vi "test_easy_spline_fft.vi"() -> ()   [LabVIEW 2009]
doc: "Copyright (c) 2010 Stepan A. Baranov (stepan@baranov.su)\nAll rights reserved.\nweb-site: www.OCTLab.org"
uses:
  <vilib>/Analysis/4window.llb/Hanning Window (DBL).vi
  <vilib>/Analysis/NI_AALPro.lvlib
  OCTLib_64.dll
panel:
  out "error out":errorcluster
  out "Im part":dbl[](array[numeric])
  out "Re part":dbl[](array[numeric])
  out "Phase A-scan":dbl[](array[numeric])
  out "Intensity A-scan":dbl[](array[numeric])
  out "Im":dbl[](array[numeric])
  out "Re":dbl[](array[numeric])
  out "phase":dbl[](array[numeric])
  out "intensity":dbl[](array[numeric])
  out "time for FFT":u32
  in  "RSM_STAT?":bool=TRUE
  in  "stop":bool
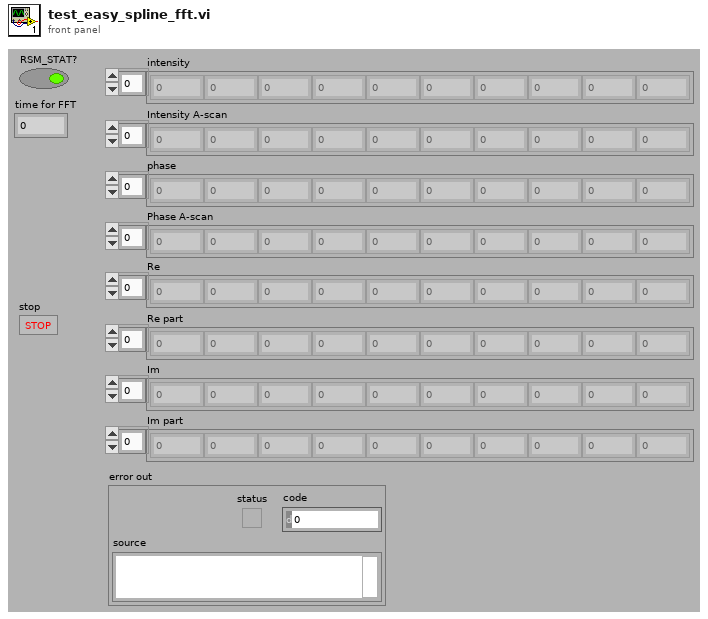
[diagram p1: front panel]
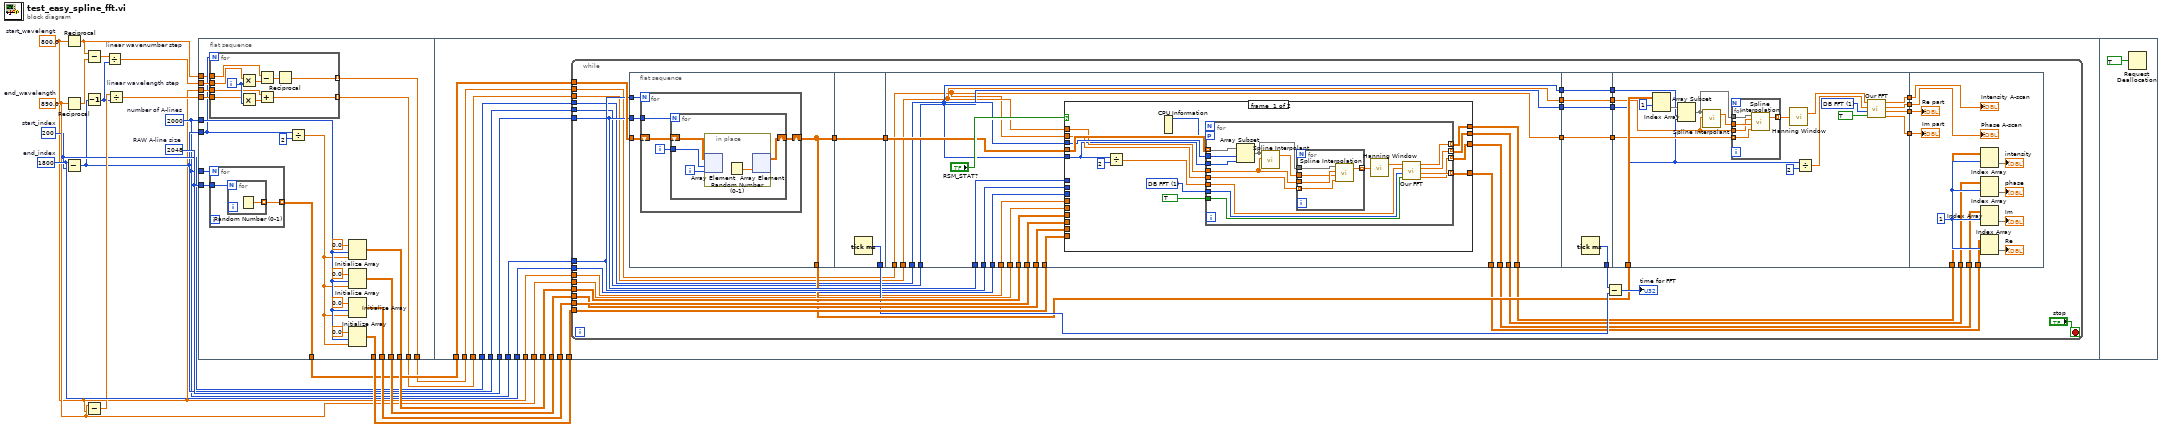
[diagram p0: block diagram]
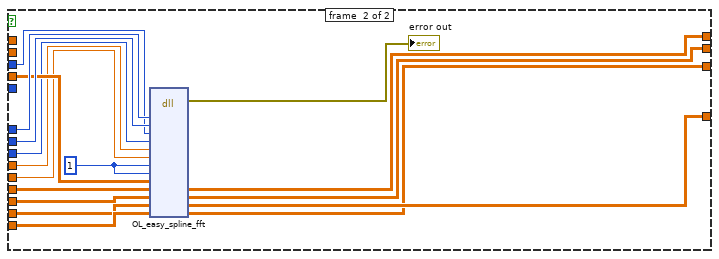
[diagram p2: hidden frame]
diagram:
  w1 = 800.0  # start_wavelengt
  w9 = 890.0  # end_wavelength
  w15 = 1800  # end_index
  w8 = 200  # start_index
  w4 = 2000  # number of A-lines
  w16 = 2048  # RAW A-line size
  n1 = Reciprocal(x=w1) -> (1/x=w2:dbl)
  n2 = Reciprocal(x=w9) -> (1/x=w3:dbl)
  n3 = Subtract(x=w15, y=w8) -> (x-y=w7:i32)
  n4 = Subtract(x=w2, y=w3) -> (x-y=w13:dbl)
  n5 = Decrement(x=w7) -> (x-1=w12:i32)
  n6 = Subtract(x=w9, y=w1) -> (x-y=w14:dbl)
  n7 = Divide "linear wavenumber step"(x=w13, y=w12) -> (x/y=w11:dbl)
  n8 = Divide "linear wavelength step"(x=w14, y=w12) -> (x/y=w10:dbl)
  n9 = flat-sequence {
    tunnel: w16 -> [w42]
    tunnel: w4 -> [w41]
    tunnel: w4 -> [w36]
    tunnel: [w35] -> w21
    tunnel: [w34] -> w20
    tunnel: [w33] -> w19
    tunnel: [w32] -> w18
    tunnel: [w31] -> w17
    tunnel: w7 -> [w25]
    tunnel: w11 -> [w30]
    tunnel: w10 -> [w29]
    tunnel: w1 -> [w28]
    tunnel: [w27] -> w6
    tunnel: [w26] -> w5
    tunnel: w2 -> [w22]
    tunnel: w4 -> [w69]
    tunnel: w16 -> [w68]
    tunnel: w21 -> [w67]
    tunnel: w20 -> [w66]
    tunnel: w19 -> [w65]
    tunnel: w18 -> [w64]
    tunnel: w17 -> [w63]
    tunnel: w8 -> [w62]
    tunnel: w15 -> [w61]
    tunnel: w1 -> [w60]
    tunnel: w9 -> [w59]
    tunnel: w7 -> [w58]
    tunnel: w6 -> [w57]
    tunnel: w5 -> [w56]
    frame #0 {
      n10 = for {
        N: w25 -> [_]
        tunnel: w30 -> [w52]
        tunnel: [w44] -> w26 mode=indexing
        tunnel: w29 -> [w49]
        tunnel: w28 -> [w48]
        tunnel: [w43] -> w27 mode=indexing
        tunnel: w22 -> [w46]
        i -> [w50]
        n11 = Multiply(x=w52, y=w50) -> (x*y=w51:dbl)
        n12 = Multiply(x=w49, y=w50) -> (x*y=w47:dbl)
        n13 = Subtract(x=w46, y=w51) -> (x-y=w45:dbl)
        n14 = Add(x=w48, y=w47) -> (x+y=w43:dbl)
        n15 = Reciprocal(x=w45) -> (1/x=w44:dbl)
      }
      n16 = for {
        N: w41 -> [_]
        tunnel: [w54] -> w31 mode=indexing
        tunnel: w42 -> [w53]
        n17 = for {
          N: w53 -> [_]
          tunnel: [w55] -> w54 mode=indexing
          n18 = Random Number (0-1)() -> (number: 0 to 1=w55:dbl)
        }
      }
      n19 = Divide(x=w25, y=2) -> (x/y=w23:dbl)
      n20 = Initialize Array(0.0 ("element"), w36, w23) -> (w34:dbl[][])
      n21 = Initialize Array(0.0 ("element"), w36, w23) -> (w33:dbl[][])
      n22 = Initialize Array(0.0 ("element"), w36, w23) -> (w35:dbl[][])
      n23 = Initialize Array(0.0 ("element"), w36, w23) -> (w32:dbl[][])
    }
    frame #1 {
      n24 = while {
        tunnel: w63 -> [w105]
        tunnel: w69 -> [w97]
        tunnel: w68 -> [w96]
        tunnel: w67 -> [w104]
        tunnel: w66 -> [w103]
        tunnel: w65 -> [w102]
        tunnel: w64 -> [w101]
        tunnel: w62 -> [w84]
        tunnel: w61 -> [w83]
        tunnel: w60 -> [w82]
        tunnel: w59 -> [w81]
        tunnel: w58 -> [w80]
        tunnel: w57 -> [w79]
        tunnel: w56 -> [w78]
        stop <- "stop" stop-if-true
        n25 = flat-sequence {
          tunnel: w105 -> [w110]
          tunnel: w97 -> [w109]
          tunnel: w96 -> [w108]
          tunnel: [w107] -> w95
          tunnel: [w107] -> w85
          tunnel: [w121] -> w100
          tunnel: [w120] -> w86
          tunnel: w85 -> [w120]
          tunnel: w104 -> [w139]
          tunnel: w103 -> [w138]
          tunnel: w102 -> [w137]
          tunnel: w101 -> [w136]
          tunnel: w96 -> [w135]
          tunnel: w97 -> [w134]
          tunnel: [w133] -> w90
          tunnel: [w132] -> w89
          tunnel: [w131] -> w88
          tunnel: [w130] -> w87
          tunnel: w86 -> [w129]
          tunnel: w84 -> [w125]
          tunnel: w83 -> [w128]
          tunnel: w82 -> [w127]
          tunnel: w81 -> [w126]
          tunnel: w80 -> [w124]
          tunnel: w79 -> [w123]
          tunnel: w78 -> [w122]
          tunnel: [w125] -> w76
          tunnel: [w124] -> w74
          tunnel: [w123] -> w73
          tunnel: [w122] -> w70
          tunnel: [w197] -> w98
          tunnel: [w196] -> w77
          tunnel: w76 -> [w196]
          tunnel: [w195] -> w75
          tunnel: w74 -> [w195]
          tunnel: w73 -> [w194]
          tunnel: [w194] -> w72
          tunnel: [w193] -> w71
          tunnel: w70 -> [w193]
          tunnel: w95 -> [w216]
          tunnel: [w211] -> w94
          tunnel: [w210] -> w93
          tunnel: [w209] -> w92
          tunnel: [w208] -> w91
          tunnel: w77 -> [w205]
          tunnel: w75 -> [w200]
          tunnel: w72 -> [w203]
          tunnel: w71 -> [w202]
          tunnel: w94 -> [w234]
          tunnel: w93 -> [w233]
          tunnel: w92 -> [w232]
          tunnel: w91 -> [w231]
          tunnel: w90 -> [w229]
          tunnel: w89 -> [w227]
          tunnel: w88 -> [w225]
          tunnel: w87 -> [w223]
          frame #0 {
            n26 = for {
              N: w109 -> [_]
              shift-right: [w112] -> w107
              shift-left: w110 -> [w113]
              tunnel: w108 -> [w114]
              i -> [w111]
              n27 = for {
                N: w114 -> [_]
                shift-right: [w115] -> w112
                shift-left: w113 -> [w118]
                tunnel: w111 -> [w117]
                i -> [w116]
                n28 = in-place {
                  n29 = in-place-array #1(w118, w117, w116) -> ()  [unwired: 1 out]
                  n30 = Random Number (0-1)() -> (number: 0 to 1=w119:dbl)
                  n31 = in-place-array #1(w119) -> (w115:dbl[][])  [unwired: 2 out]
                }
              }
            }
          }
          frame #1 {
            n32 = Tick Count (ms)() -> (millisecond timer value=w121:u32)
          }
          frame #2 {
            n33 = case shown="True" "RSM_STAT?" {
              tunnel: w139 -> [_ w189]
              tunnel: w138 -> [_ w192]
              tunnel: w137 -> [_ w191]
              tunnel: w136 -> [_ w190]
              tunnel: w135 -> [_ w188]
              tunnel: w134 -> [_ w187]
              tunnel: w129 -> [w154 w185]
              tunnel: [w150 w184] -> w133
              tunnel: [w149 w183] -> w132
              tunnel: [w148 w182] -> w131
              tunnel: [w147 w181] -> w130
              tunnel: w125 -> [w146 w180]
              tunnel: w128 -> [_ w179]
              tunnel: w127 -> [_ w178]
              tunnel: w126 -> [_ w177]
              tunnel: w124 -> [w143 _]
              tunnel: w123 -> [w145 _]
              tunnel: w122 -> [w144 _]
              frame #0 {
                w151 = 1 items=["LINEAR FFT", "DB FFT"] ("A-scan type")
                n34 = Divide(x=w143, y=2) -> (x/y=w141:dbl)
                n35 = CPU Information() -> (4:w153:i32)  [unwired: 3 out]
                n36 = for {
                  workers-P: w153 -> [_]
                  tunnel: [w169] -> w150 mode=indexing
                  tunnel: [w168] -> w149 mode=indexing
                  tunnel: [w167] -> w148 mode=indexing
                  tunnel: [w166] -> w147 mode=indexing
                  tunnel: w154 -> [w163] mode=indexing
                  tunnel: TRUE ("need phase?") -> [w165]
                  tunnel: w151 -> [w164]
                  tunnel: w146 -> [w162]
                  tunnel: w143 -> [w161]
                  tunnel: w145 -> [w158]
                  tunnel: w144 -> [w160]
                  tunnel: w141 -> [w155]
                  n37 = Array Subset(array=w163, index=w162, length=w161) -> (w159:dbl[])
                  n38 = call <vilib>:"Spline Interpolant.vi"("X"=w158, "Y"=w159) -> ("Interpolant"=w157:dbl[])  [unwired: 2 in, 1 out]
                  n39 = for {
                    tunnel: w160 -> [w172] mode=indexing
                    tunnel: w159 -> [w175]
                    tunnel: w158 -> [w174]
                    tunnel: w157 -> [w173]
                    tunnel: [w171] -> w156 mode=indexing
                    n40 = call <vilib>:"Spline Interpolation.vi"("x value"=w172, "Interpolant"=w173, "X"=w174, "Y"=w175) -> ("interpolation value"=w171:dbl)  [unwired: 1 out]
                  }
                  n41 = call-poly <vilib>:"Hanning Window.vi"("X"=w156) -> ("Windowed X"=w170:dbl[])  [unwired: 1 out]
                  n42 = call "Our FFT.vi"("need phase?"=w165, "A-scan type"=w164, "FFT A-scan size"=w155, "RAW A-line"=w170) -> ("Im part"=w166:dbl[], "Re part"=w167:dbl[], "Phase A-scan"=w168:dbl[], "Intensity A-scan"=w169:dbl[])
                }
              }
              frame #1 {
                w186 = i8 1 ("hanning_flag")
                n43 = dll-call lib="OCTLib**.*" fn="OL_easy_spline_fft"("width"=w188, "height"=w187, "start_index"=w180, "end_index"=w179, "start_wavelengt"=w178, "end_wavelength"=w177, "hanning_flag"=w186, "log10_flag"=w186, "input"=w185, "intensity"=w192, "phase"=w191, "Re"=w189, "Im"=w190) -> (error out=→"error out":errorcluster, "intensity"=w184:dbl[][], "phase"=w183:dbl[][], "Re"=w182:dbl[][], "Im"=w181:dbl[][])  [unwired: 13 in, 1 out]
              }
            }
          }
          frame #3 {
            n44 = Tick Count (ms)() -> (millisecond timer value=w197:u32)
          }
          frame #4 {
            w213 = 1 items=["LINEAR FFT", "DB FFT"] ("A-scan type")
            n45 = Index Array(array=w216, index (row)=1) -> (element=w206:dbl[])  [unwired: 1 in]
            n46 = Array Subset(array=w206, index=w205, length=w200) -> (w204:dbl[])
            n47 = call <vilib>:"Spline Interpolant.vi"("X"=w203, "Y"=w204) -> ("Interpolant"=w207:dbl[])  [unwired: 2 in, 1 out]
            n48 = for {
              tunnel: w207 -> [w221]
              tunnel: w204 -> [w220]
              tunnel: w203 -> [w219]
              tunnel: w202 -> [w218] mode=indexing
              tunnel: [w217] -> w201 mode=indexing
              n49 = call <vilib>:"Spline Interpolation.vi"("x value"=w218, "Interpolant"=w221, "X"=w219, "Y"=w220) -> ("interpolation value"=w217:dbl)  [unwired: 1 out]
            }
            n50 = call-poly <vilib>:"Hanning Window.vi"("X"=w201) -> ("Windowed X"=w214:dbl[])  [unwired: 1 out]
            n51 = Divide(x=w200, y=2) -> (x/y=w198:dbl)
            n52 = call "Our FFT.vi"("need phase?"=TRUE, "A-scan type"=w213, "FFT A-scan size"=w198, "RAW A-line"=w214) -> ("Im part"=w208:dbl[], "Re part"=w209:dbl[], "Phase A-scan"=w210:dbl[], "Intensity A-scan"=w211:dbl[])
          }
          frame #5 {
            w230 = 1 ("index (row)")
            n53 = Index Array(array=w229, index (row)=w230) -> (element=→"intensity":dbl[])  [unwired: 1 in]
            n54 = Index Array(array=w227, index (row)=w230) -> (element=→"phase":dbl[])  [unwired: 1 in]
            n55 = Index Array(array=w223, index (row)=w230) -> (element=→"Im":dbl[])  [unwired: 1 in]
            n56 = Index Array(array=w225, index (row)=w230) -> (element=→"Re":dbl[])  [unwired: 1 in]
            "Intensity A-scan" <- w234
            "Phase A-scan" <- w233
            "Re part" <- w232
            "Im part" <- w231
          }
        }
        n57 = Subtract(x=w98, y=w100) -> (x-y=→"time for FFT":u32)
      }
    }
    frame #2 {
      n58 = Request Deallocation(TRUE ("flag")) -> ()
    }
  }
